vi "Abort Session.vi"(0 "instrument handle":refnum<k15>[](array[refnum]), 2 "Software Flags":T1, 7 "channel name":string[](array[string]), 11 "error in (no error)":errorcluster) -> (15 "error out":errorcluster)   [LabVIEW 2024, in "devicePowerSequencerCoreLogic.lvlib"]
uses:
  devicePowerSequencerCoreLogic.lvlib
  controls/Software Flags.ctl
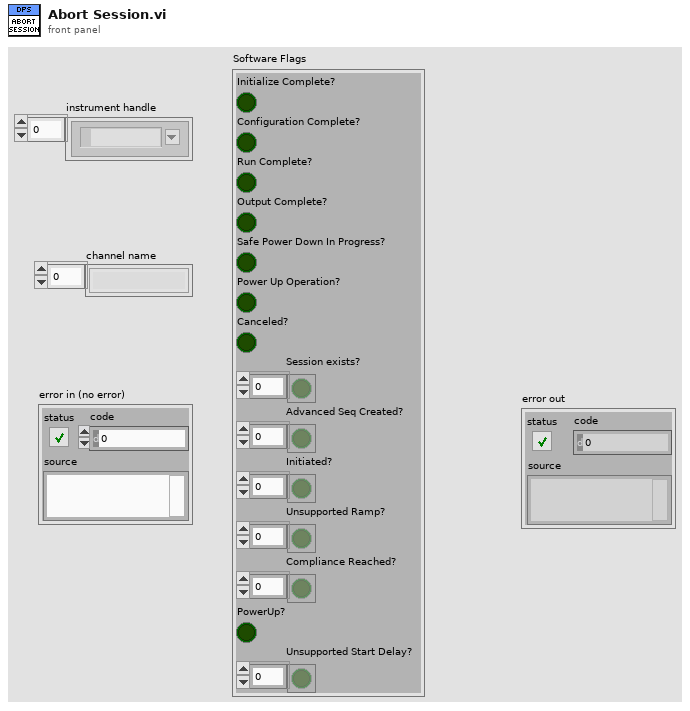
[diagram p1: front panel]
types:
  T1 = typedef "devicePowerSequencerCoreLogic.lvlib/Software Flags.ctl" = cluster{"Initialize Complete?":bool, "Configuration Complete?":bool, "Run Complete?":bool, "Output Complete?":bool, "Safe Power Down In Progress?":bool, "Power Up Operation?":bool, "Canceled?":bool, "Session exists?":bool[], "Advanced Seq Created?":bool[], "Initiated?":bool[], "Unsupported Ramp?":bool[], "Compliance Reached?":bool[], "PowerUp?":bool, "Unsupported Start Delay?":bool[]}
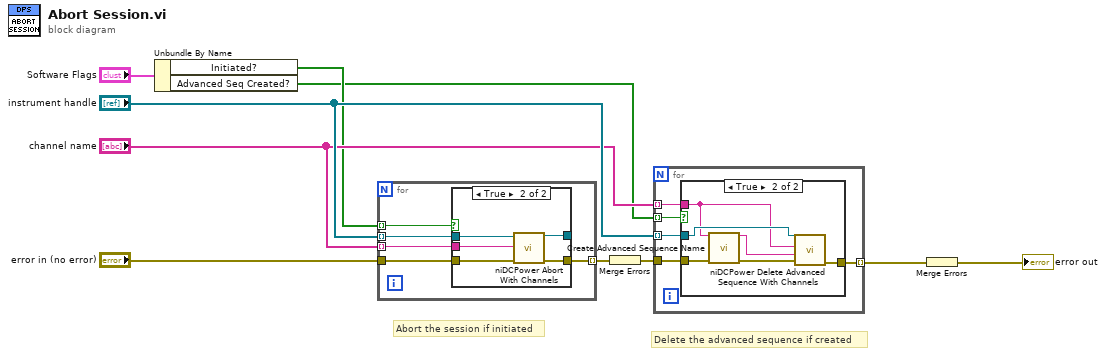
[diagram p0: block diagram]
diagram:
  # "Delete the advanced sequence if created"
  # "Abort the session if initiated"
  n1 = Unbundle By Name("Software Flags") -> ("Initiated?"=w5:bool[], "Advanced Seq Created?"=w4:bool[])
  n2 = for {
    tunnel: "error in (no error)" -> [w15]
    tunnel: "instrument handle" -> [w14] mode=indexing
    tunnel: "channel name" -> [w13] mode=indexing
    tunnel: [w12] -> w3 mode=indexing
    tunnel: w5 -> [w11] mode=indexing
    n3 = case shown="True" w11 {
      tunnel: w15 -> [w16 w22]
      tunnel: w14 -> [w17 w21]
      tunnel: w13 -> [_ w20]
      tunnel: [w17 w19] -> _
      tunnel: [w16 w18] -> w12
      frame False {
      }
      frame True {
        n4 = call <instrlib>:"niDCPower Abort With Channels.vi"("error in (no error)"=w22, "channel name"=w20, "instrument handle"=w21) -> ("error out"=w18:errorcluster, "instrument handle out"=w19:refnum<k15>)  [unwired: 7 in]
      }
    }
  }
  n5 = Merge Errors(w3) -> (w2:errorcluster)
  n6 = for {
    tunnel: "instrument handle" -> [w27] mode=indexing
    tunnel: w2 -> [w26]
    tunnel: w4 -> [w25] mode=indexing
    tunnel: "channel name" -> [w24] mode=indexing
    tunnel: [w23] -> w1 mode=indexing
    n7 = case shown="True" w25 {
      tunnel: [w28 w34] -> w23
      tunnel: w27 -> [_ w30]
      tunnel: w26 -> [w28 w33]
      tunnel: w24 -> [_ w29]
      frame False {
      }
      frame True {
        n8 = call "Create Advanced Sequence Name.vi"("Channel Name"=w29, "error in (no error)"=w33) -> ("String"=w32:string, "error out"=w31:errorcluster)  [unwired: 12 in]
        n9 = call <instrlib>:"niDCPower Delete Advanced Sequence With Channels.vi"("error in (no error)"=w31, "sequence name"=w32, "channel name"=w29, "instrument handle"=w30) -> ("error out"=w34:errorcluster)  [unwired: 6 in, 1 out]
      }
    }
  }
  n10 = Merge Errors(w1) -> (→"error out":errorcluster)
